vi "TX ADU.vi"(8 "error in (no error)":errorcluster, 9 "PDU_req in":T1={"Function Code"=1, "Data"=[], "RTU_DataBytes"=0}, 11 "MB_ADU_TCP in":refnum<class "MB_ADU_TCP.lvclass">) -> (0 "error out":errorcluster, 1 "TX Data":string, 3 "MB_ADU_TCP out":refnum<class "MB_ADU_TCP.lvclass">)   [LabVIEW 2016, in "MB Master.lvlib" / "MB_ADU_TCP.lvclass"]
doc: "Defines the transmit procedure for a Modbus TCP ADU. The PDU to be transmitted should be written to PDU_req prior to calling this VI."
uses:
  MB_ADU_TCP.lvclass
  C:/Users/illogicdev/Desktop/IGUS/20190906-1xdryveD1+LABview+ModbusTCP(Gateway)/IgusPositioningSystem Folder/Modules/Libraries/Modbus-Master/MB_ADU/MB_ADU.lvclass
  MB_PDU/MB_PDU_Cluster.ctl
  MB_ADU_TCP.lvclass/MB_ADU_TCP.ctl
  MB_ADU/MB_ADU.lvclass/MB_ADU.ctl
  MB_ADU/Read Slave ID.vi
  MB_ADU/Write TX Data.vi
  MB_ADU/Write TX Timestamp.vi
  MB Master.lvlib
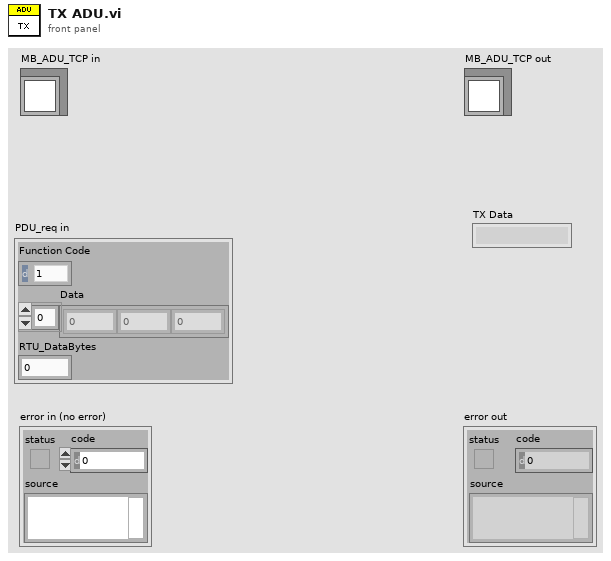
[diagram p1: front panel]
types:
  T1 = typedef "MB Master.lvlib/MB_PDU_Cluster.ctl" = cluster{"Function Code":u8, "Data":u8[], "RTU_DataBytes":i32}
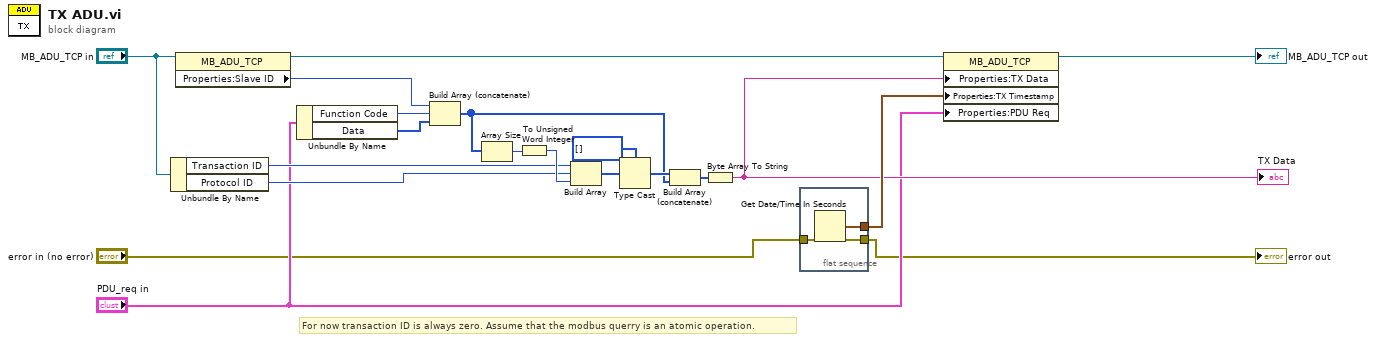
[diagram p0: block diagram]
diagram:
  # "For now transaction ID is always zero. Assume that the modbus querry is an atomic operation."
  n1 = Unbundle By Name("MB_ADU_TCP in") -> ("Transaction ID"=w8:u16, "Protocol ID"=w7:u16)
  n2 = property class="MB_ADU_TCP"(reference="MB_ADU_TCP in") -> (reference out=w20:refnum<class "MB_ADU_TCP.lvclass">, "Properties:Slave ID"=w18:u8)  [unwired: 1 in, 1 out]
  n3 = Unbundle By Name("PDU_req in") -> ("Function Code"=w5:u8, "Data"=w4:u8[])
  n4 = Build Array (concatenate)(w18, w5, w4) -> (w12:u8[])
  n5 = Array Size(array=w12) -> (size(s)=w17:i32)
  n6 = To Unsigned Word Integer(number=w17) -> (unsigned 16bit integer=w16:u16)
  n7 = Build Array(w8, w7, w16) -> (w15:u16[])
  n8 = Type Cast(type=u8[] [], x=w15) -> (*(type *) &x=w13:u8[])
  n9 = Build Array (concatenate)(w13, w12) -> (w11:u8[])
  n10 = Byte Array To String(unsigned byte array=w11) -> (string=w6:string)
  "TX Data" <- w6
  n11 = flat-sequence {
    tunnel: "error in (no error)" -> [w22]
    tunnel: [w22] -> w2
    tunnel: [w21] -> w10
    frame #0 {
      n12 = Get Date/Time In Seconds() -> (seconds since 1Jan1904=w21:timestamp)
    }
  }
  n13 = property class="MB_ADU_TCP"(reference=w20, "Properties:TX Data"=w6, "Properties:TX Timestamp"=w10, "Properties:PDU Req"="PDU_req in") -> (reference out=→"MB_ADU_TCP out":refnum<class "MB_ADU_TCP.lvclass">)  [unwired: 1 in, 1 out]
  "error out" <- w2
